vi "Connect.vi"(8 "error in (no error)":errorcluster, 11 "TcpReader in":refnum<class "TcpReader.lvclass">) -> (0 "error out":errorcluster, 3 "TcpReader out":refnum<class "TcpReader.lvclass">)   [LabVIEW 2013, in "TcpReader.lvclass"]
doc: "Opens a TCP connection"
uses:
  TcpReader.lvclass
  TcpReader.lvclass/TcpReader.ctl
  Interface/TCP/TCP/TCP.lvclass
  Interface/TCP/TCP/TCP Open (port).vi
  Interface/TCP/TCP/TCP Open (name).vi
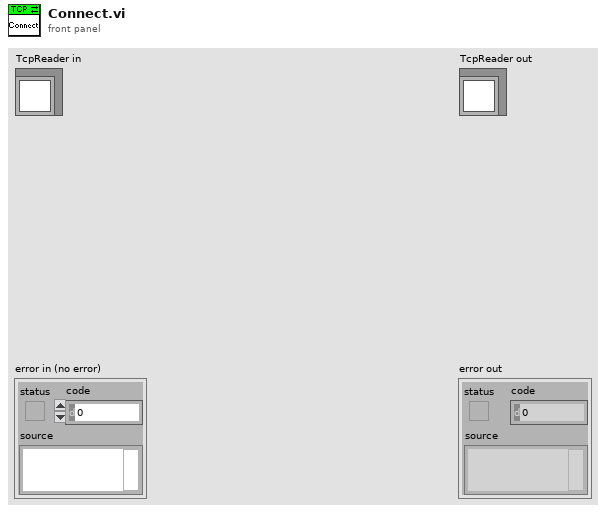
[diagram p1: front panel]
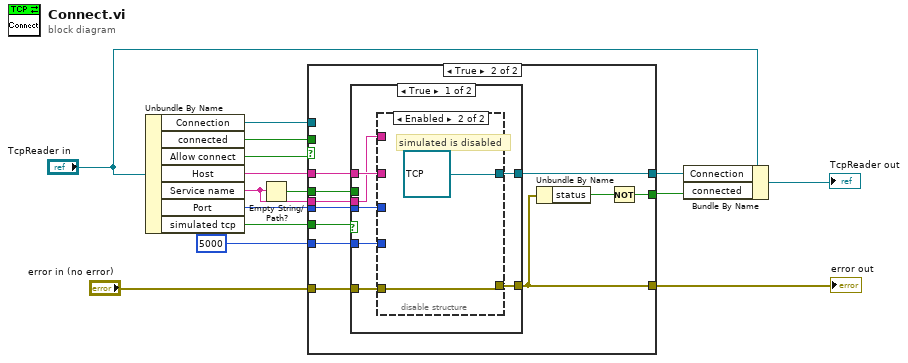
[diagram p0: block diagram]
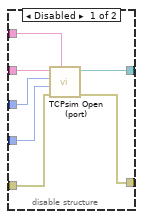
[diagram p3: hidden frame]
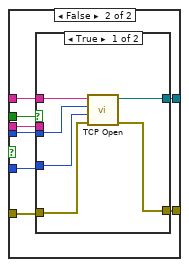
[diagram p4: hidden frame]
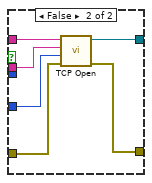
[diagram p5: hidden frame]
diagram:
  n1 = Unbundle By Name("TcpReader in") -> ("Connection"=w3:refnum<class "TCP.lvclass">, "connected"=w2:bool, "Allow connect"=w4:bool, "Host"=w9:string, "Service name"=w6:string, "Port"=w7:u16, "simulated tcp"=w1:bool)
  n2 = Empty String/Path?(string/path=w6) -> (empty?=w8:bool)
  n3 = case shown="True" w4 {
    tunnel: 5000 ("timeout ms (60000)") -> [_ w29]
    tunnel: [w18 w28] -> w10
    tunnel: w9 -> [_ w27]
    tunnel: w8 -> [_ w26]
    tunnel: w7 -> [_ w25]
    tunnel: w6 -> [_ w24]
    tunnel: "error in (no error)" -> [w16 w23]
    tunnel: [w16 w22] -> w12
    tunnel: [w17 w20] -> w5
    tunnel: w3 -> [w18 _]
    tunnel: w2 -> [w17 _]
    tunnel: w1 -> [_ w19]
    frame False {
    }
    frame True {
      n4 = case shown="True" w19 {
        tunnel: w29 -> [w33 w53]
        tunnel: [w36 w52] -> w28
        tunnel: w27 -> [w35 w51]
        tunnel: w26 -> [_ w50]
        tunnel: w25 -> [w34 w49]
        tunnel: w24 -> [w32 w48]
        tunnel: w23 -> [w30 w47]
        tunnel: [w31 w46] -> w22
        frame True {
          n5 = disable-structure shown="Enabled" {
            disable-tunnel: [w43 refnum<class "TCP.lvclass"> refnum ("Connection")] -> w36
            disable-tunnel: w35 -> [w42 _]
            disable-tunnel: w34 -> [w41 _]
            disable-tunnel: w33 -> [w40 _]
            disable-tunnel: w32 -> [w39 _]
            disable-tunnel: [w38 w45] -> w31
            disable-tunnel: w30 -> [w37 w45]
            frame Disabled {
              n6 = call "TCPsim Open (port).vi"("device name"=w39, "error in (no error)"=w37, "timeout ms (60000)"=w40, "remote port"=w41, "address"=w42) -> ("error out"=w38:errorcluster, "TCPsimulated out"=w43:refnum<class "TCPsimulated.lvclass">)  [unwired: 5 in]
            }
            frame Enabled {
              # "simulated is disabled"
            }
          }
        }
        frame False {
          n7 = case shown="True" w50 {
            tunnel: w53 -> [w59 w65]
            tunnel: [w58 w64] -> w52
            tunnel: w51 -> [w57 w63]
            tunnel: w49 -> [w56 _]
            tunnel: w48 -> [_ w62]
            tunnel: w47 -> [w55 w61]
            tunnel: [w54 w60] -> w46
            frame True {
              n8 = call-poly "TCP Open.vi"("error in (no error)"=w55, "timeout ms (60000)"=w59, "remote port or service name"=w56, "address"=w57) -> ("error out"=w54:errorcluster, "TCP out"=w58:refnum<class "TCP.lvclass">)  [unwired: 6 in]
            }
            frame False {
              n9 = call-poly "TCP Open.vi"("error in (no error)"=w61, "timeout ms (60000)"=w65, "remote port or service name"=w62, "address"=w63) -> ("error out"=w60:errorcluster, "TCP out"=w64:refnum<class "TCP.lvclass">)  [unwired: 6 in]
            }
          }
        }
      }
      n10 = Unbundle By Name(w22) -> ("status"=w21:bool)
      n11 = Not(x=w21) -> (.not. x?=w20:bool)
    }
  }
  "error out" <- w12
  n12 = Bundle By Name(cluster="TcpReader in", "Connection"=w10, "connected"=w5) -> (→"TcpReader out":refnum<class "TcpReader.lvclass">)
